vi "VMI_acquire_rewrite_get_loop_working.vi"(4 "Big_image Array":i16[][][](array[numeric]), 5 "Peak Find Settings":T2, 6 "Collect_refs":T1, 7 "Queue Array":T4[](array[typedef]), 8 "error in":errorcluster, 9 "Collection Information":T3[](array[typedef]), 10 "Camera Session":T5, 11 "IMAQ In":T6) -> (0 "error IO":errorcluster, 2 "Peak Array":cluster{"X":sgl, "Y":sgl}[][](array[cluster]), 3 "Histogram":i32[][](array[numeric]))   [LabVIEW 2015]
uses:
  <vilib>/vision/Image Controls.llb/IMAQ Image.ctl
  <vilib>/userdefined/High Color/IMAQdx.ctl
  Type defs/FileAcq_v1_Ctrl.ctl
  Type defs/VMI_collection_refs.ctl
  Array_subVIs/Merge_into_Array.vi
  Array_subVIs/Merge_into_Array_cluster.vi
panel:
  out "xaxis":i32[][](array[numeric])
  out "XY Graph":cluster{"Y":dbl[], "Y":dbl[]}[](graph)
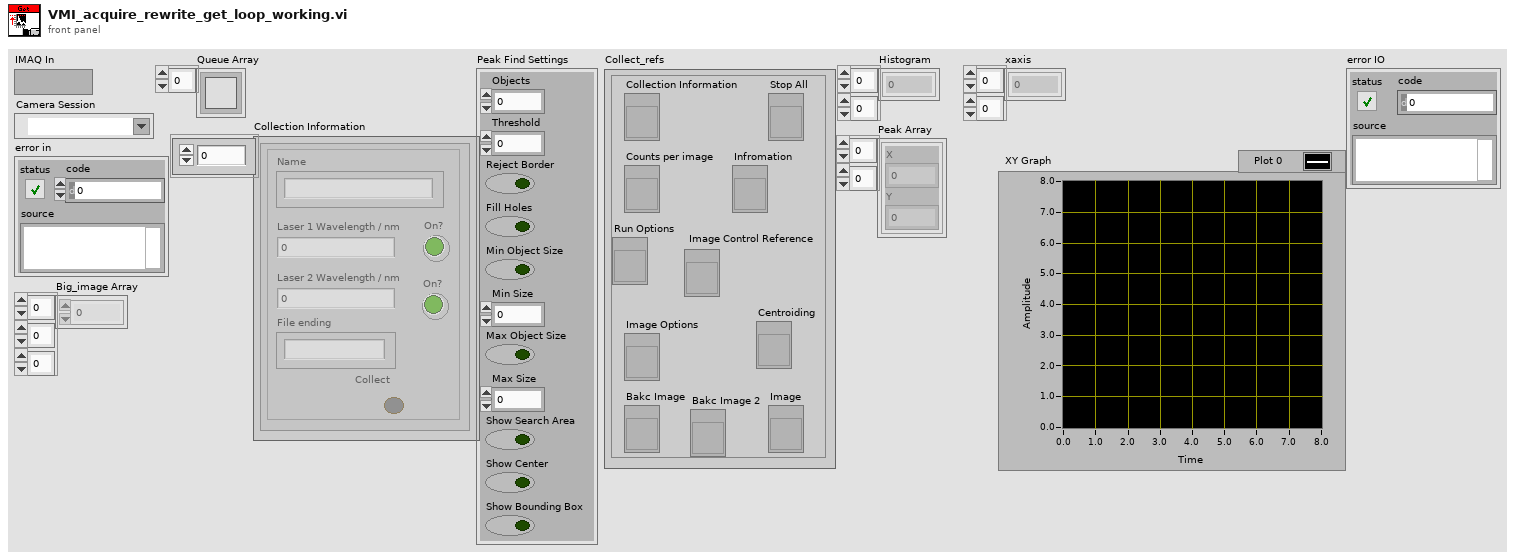
[diagram p1: front panel]
types:
  T1 = typedef "VMI_collection_refs.ctl" = cluster{"Stop All":refnum<vi>, "Collection Information ":refnum<vi>, "Infromation":refnum<vi>, "Counts per image":refnum<vi>, " Image Control Reference ":refnum<vi>, "Run Options":refnum<vi>, "Image Options":refnum<vi>, "Centroiding":refnum<vi>, "Image":refnum<vi>, "Bakc Image":refnum<vi>, "Bakc Image 2":refnum<vi>}
  T2 = cluster{"Objects":u16, "Threshold":i32, "Reject Border":bool, "Fill Holes":bool, "Min Object Size":bool, "Min Size":i32, "Max Object Size":bool, "Max Size":i32, "Show Search Area":bool, "Show Center":bool, "Show Bounding Box":bool}
  T3 = typedef "FileAcq_v1_Ctrl.ctl" = cluster{"Type":string, "LaserWave1":dbl, "Shutter1":bool, "LaserWave2":dbl, "Shutter2":bool, "FileEnd":string, "Collect":bool}
  T4 = typedef "Queue RefNum" = refnum<k1>
  T5 = typedef "IMAQdx.ctl" = refnum<k21>
  T6 = typedef "IMAQ Image.ctl" = refnum<image>
  T7 = cluster{"Total Time / ms":dbl, "Image Total Collection Time":dbl, "Image Loop time / ms":dbl, "Peak Total Find Time":dbl, "Peak Find Time / ms":dbl, "Camera Rate / Hz":dbl, "Total Number of Loops":dbl, "Current Loop Number":dbl, "Number of Image Loops":dbl, "Run Mode":dbl}
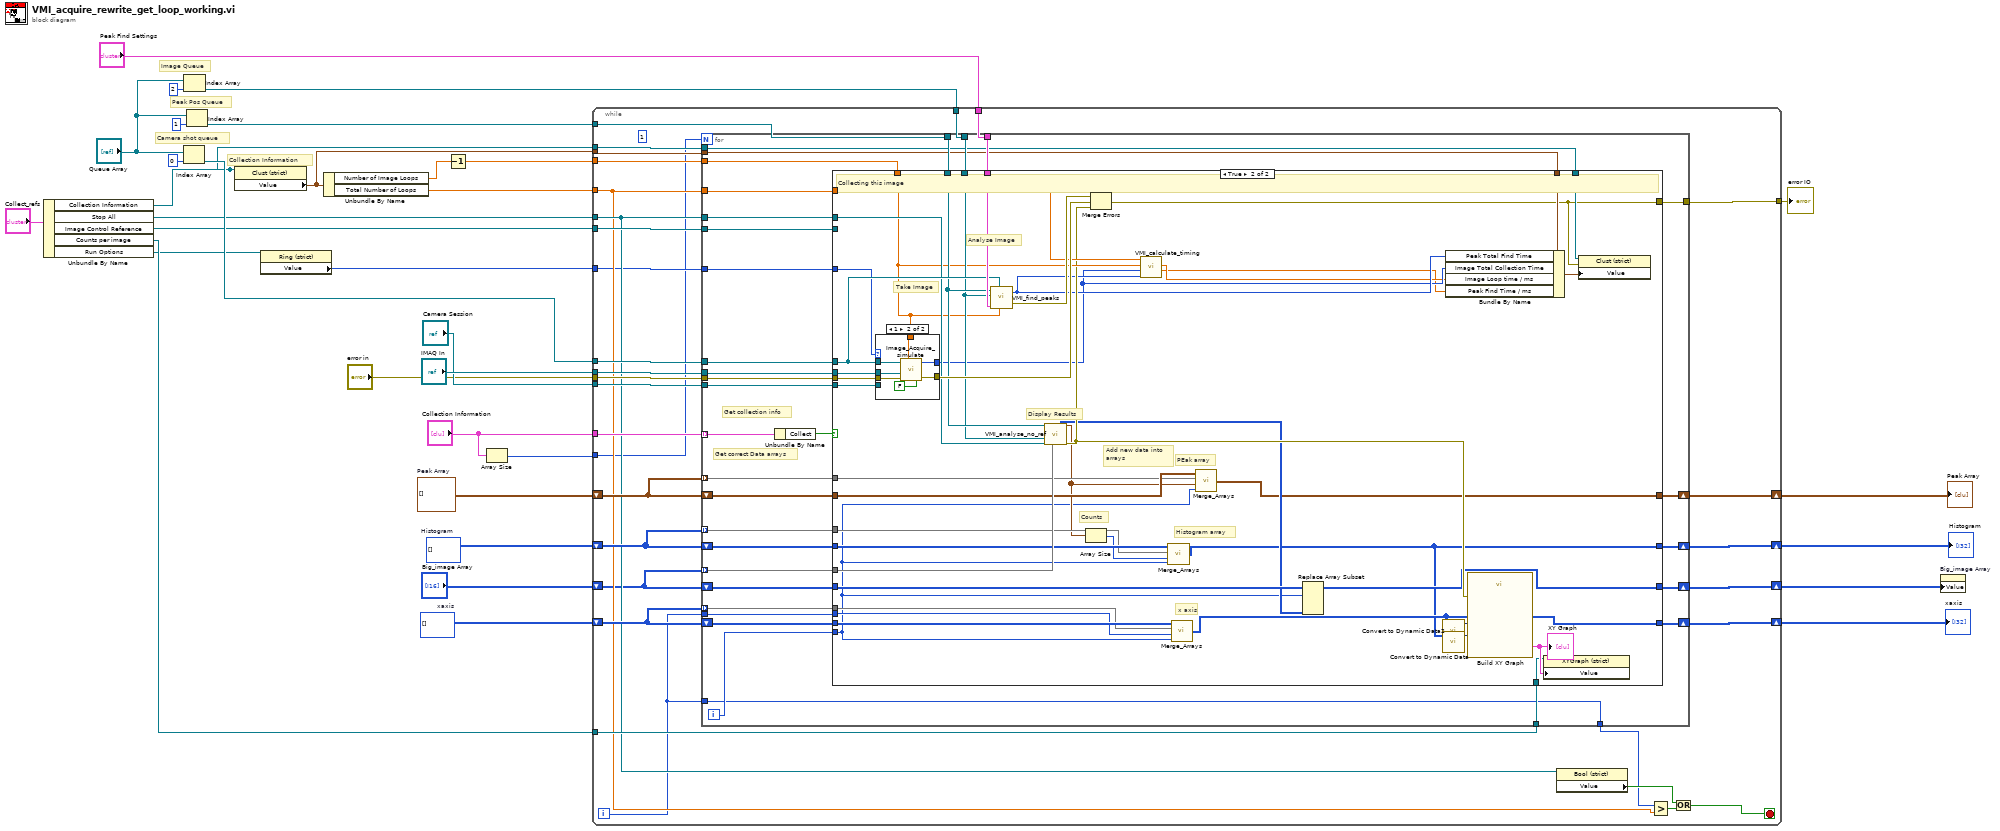
[diagram p0: block diagram]
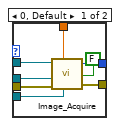
[diagram p3: hidden frame]
diagram:
  w11 = i32[][] []  # xaxis
  w9 = i32[][] []  # Histogram
  w12 = cluster{"X":sgl, "Y":sgl}[][] []  # Peak Array
  # "Collection Information"
  # "Image Queue"
  # "Peak Pos Queue"
  # "Camera shot queue"
  n1 = Unbundle By Name("Collect_refs") -> ("Collection Information"=w14:refnum<vi>, "Stop All"=w20:refnum<vi>, "Image Control Reference"=w19:refnum<vi>, "Counts per image"=w10:refnum<vi>, "Run Options"=w2:refnum<vi>)
  n2 = Index Array(array="Queue Array", index=0) -> (element=w29:T4)
  n3 = Index Array(array="Queue Array", index=2) -> (element=w22:T4)
  n4 = Index Array(array="Queue Array", index=1) -> (element=w25:T4)
  n5 = property class="Clust (strict)"(reference=w14) -> ("Value"=w15:T7)  [unwired: 1 in, 2 out]
  n6 = property class="Ring (strict)"(reference=w2) -> ("Value"=w1:u16)  [unwired: 1 in, 2 out]
  n7 = Unbundle By Name(w15) -> ("Number of Image Loops"=w18:dbl, "Total Number of Loops"=w16:dbl)
  n8 = Decrement(x=w18) -> (x-1=w17:dbl)
  n9 = Array Size(array="Collection Information") -> (size(s)=w13:i32)
  n10 = while {
    tunnel: "IMAQ In" -> [w64]
    tunnel: "Camera Session" -> [w63]
    tunnel: "error in" -> [w62]
    tunnel: w29 -> [w61]
    tunnel: "Collection Information" -> [w60]
    tunnel: "Peak Find Settings" -> [w59]
    tunnel: w25 -> [w58]
    tunnel: w22 -> [w57]
    tunnel: w20 -> [w45]
    tunnel: w19 -> [w56]
    tunnel: w17 -> [w55]
    tunnel: w16 -> [w42]
    tunnel: w15 -> [w54]
    tunnel: w14 -> [w53]
    tunnel: w13 -> [w36]
    tunnel: w10 -> [w50]
    shift-right: [w49] -> w3
    shift-left: w12 -> [w52]
    shift-right: [w47] -> w4
    shift-left: w9 -> [w48]
    shift-right: [w46] -> w8
    shift-left: w11 -> [w51]
    tunnel: [w41] -> w7
    shift-right: [w40] -> w5
    shift-left: "Big_image Array" -> [w39]
    tunnel: w1 -> [w38]
    i -> [w35]
    stop <- w37 stop-if-true
    (unwired) 1
    n11 = for {
      N: w36 -> [_]
      tunnel: w64 -> [w97]
      tunnel: w63 -> [w96]
      tunnel: w62 -> [w95]
      tunnel: w61 -> [w94]
      tunnel: w60 -> [w76] mode=indexing
      tunnel: w59 -> [w92]
      tunnel: w58 -> [w91]
      tunnel: w57 -> [w90]
      tunnel: w45 -> [w89]
      tunnel: w56 -> [w88]
      tunnel: w52 -> [w80] mode=indexing
      tunnel: w55 -> [w86]
      tunnel: w42 -> [w85]
      tunnel: w35 -> [w77]
      tunnel: w51 -> [w78] mode=indexing
      tunnel: w54 -> [w84]
      tunnel: w53 -> [w83]
      tunnel: w48 -> [w79] mode=indexing
      tunnel: w50 -> [w74]
      shift-right: [w73] -> w49
      shift-left: w52 -> [w82]
      shift-right: [w87] -> w47
      shift-left: w48 -> [w72]
      shift-right: [w71] -> w46
      shift-left: w51 -> [w81]
      tunnel: [w70] -> w41
      shift-right: [w68] -> w40
      shift-left: w39 -> [w69]
      tunnel: w39 -> [w67] mode=indexing
      tunnel: w38 -> [w66]
      tunnel: [w65] -> w34
      tunnel: w35 -> [w65]
      i -> [w75]
      # "Get collection info"
      # "Get correct Data arrays"
      # "This loop collects for each required image"
      n12 = Unbundle By Name(w76) -> ("Collect"=w93:bool)
      n13 = case shown="True" w93 {
        tunnel: w97 -> [_ w145]
        tunnel: w96 -> [_ w144]
        tunnel: w95 -> [w102 w143]
        tunnel: w94 -> [_ w141]
        tunnel: w92 -> [_ w142]
        tunnel: w91 -> [_ w138]
        tunnel: w90 -> [_ w137]
        tunnel: w89 -> [_ w136]
        tunnel: w88 -> [_ _]
        tunnel: [w102 w123] -> w70
        tunnel: w80 -> [_ w107]
        tunnel: w82 -> [w101 w108]
        tunnel: [w101 w104] -> w73
        tunnel: w72 -> [w100 w112]
        tunnel: w79 -> [_ w111]
        tunnel: [w100 w109] -> w87
        tunnel: w86 -> [_ w134]
        tunnel: w85 -> [_ w135]
        tunnel: w77 -> [_ w114]
        tunnel: w78 -> [_ w115]
        tunnel: w81 -> [w99 w116]
        tunnel: [w99 w113] -> w71
        tunnel: w84 -> [_ w130]
        tunnel: w83 -> [_ w124]
        tunnel: w75 -> [_ w105]
        tunnel: w74 -> [_ w121]
        tunnel: w69 -> [w98 w119]
        tunnel: [w98 w118] -> w68
        tunnel: w67 -> [_ w120]
        tunnel: w66 -> [_ w103]
        frame False {
          # "Not collecting this image"
        }
        frame True {
          # "x axis"
          # "Histogram array"
          # "PEak array"
          # "Counts"
          # "Add new data into\narrays"
          # "Display Results"
          # "Analyse Image"
          # "Take Image"
          # "Collecting this image"
          n14 = case shown="1" w103 {
            tunnel: w145 -> [w152 w156]
            tunnel: w144 -> [w151 _]
            tunnel: w143 -> [w150 w160]
            tunnel: w141 -> [w149 w155]
            tunnel: [w148 w159] -> w139
            tunnel: w134 -> [w147 w157]
            tunnel: [w146 w158] -> w128
            frame 0, Default {
              n15 = call "Image_Acquire.vi"("Queue Ref in"=w149, "Acquire Time"=w147, "Image Out"=w152, "Session In"=w151, "error in (no error)"=w150, "Test Timing"=FALSE) -> ("Loop Time Out"=w146:i64, "error out"=w148:errorcluster)  [unwired: 1 in]
            }
            frame 1 {
              n16 = call "Image_Acquire_simulate.vi"("Queue Ref in"=w155, "Acquire Time"=w157, "Image Out"=w156, "error in (no error)"=w160, "Test Timing"=FALSE) -> ("Loop Time Out"=w158:i64, "error out"=w159:errorcluster)  [unwired: 2 in]
            }
          }
          n17 = call "VMI_find_peaks.vi"("Acquire Time"=w134, "Acquire Queue In"=w141, "Peak Find Settings"=w142, "Image Queue in"=w137, "Peak Position Queue in"=w138) -> ("error out"=w140:errorcluster, "x-y"=w129:u32)  [unwired: 1 in]
          n18 = call "VMI_analyse_no_ref.vi"("Peak Position Queue in"=w138, "Image in"=w137, "Stop Button Ref"=w136, "Image_array"=w120) -> ("Image_array out"=w117:i32[][], "Peaks Position Out"=w106:cluster{"X":sgl, "Y":sgl}[], "error out"=w132:errorcluster)  [unwired: 7 in, 2 out]
          n19 = Array Size(array=w106) -> (size(s)=w110:i32)
          n20 = Merge Errors(w140, w139, w132) -> (w123:errorcluster)
          n21 = call "VMI_calculate_timing.vi"("Peakfind total time"=w129, "Camera_Total_loop time"=w128, "Number of image loops"=w134, "Total loop Number"=w135) -> ("AveragePeak find time"=w126:dbl, "Average Image Loop time"=w127:dbl)  [unwired: 1 in, 1 out]
          n22 = call-poly "Merge_Arrays.vi"("Index"=w105, "Insert"=w110, "1D Array"=w111, "2D Array"=w112) -> ("Output Array"=w109:i32[][])
          n23 = call-poly "Merge_Arrays.vi"("Index"=w105, "Insert"=w114, "1D Array"=w115, "2D Array"=w116) -> ("Output Array"=w113:i32[][])
          n24 = call-poly "Merge_Arrays.vi"("Index"=w105, "1D Array Insert"=w106, "1D Array"=w107, "2D Array"=w108) -> ("Output Array"=w104:cluster{"X":sgl, "Y":sgl}[][])
          n25 = Replace Array Subset(array=w119, new element=w117, index (dim 0)=w105) -> (w118:i16[][][])  [unwired: 2 in]
          n26 = call "Convert to Dynamic Data2"("2D Array"=w113) -> ("Dynamic Data Type"=w131:dynamicdata)  [unwired: 3 in]
          n27 = call "Convert to Dynamic Data"("2D Array"=w109) -> ("Dynamic Data Type"=w133:dynamicdata)  [unwired: 3 in]
          n28 = Bundle By Name(cluster=w130, "Peak Total Find Time"=w129, "Image Total Collection Time"=w128, "Image Loop time / ms"=w127, "Peak Find Time / ms"=w126) -> (w125:T7)
          n29 = call "Build XY Graph"("error in (no error)"=w132, "Y Input"=w133, "X Input"=w131) -> ("XY Graph"=w122:cluster{"X":dbl[], "Y":dbl[]}[])  [unwired: 7 in, 1 out]
          "XY Graph" <- w122
          n30 = property on="Property Node" class="XYGraph (strict)"(reference=w121, "Value"=w122) -> ()  [unwired: 1 in, 2 out]
          n31 = property class="Clust (strict)"(reference=w124, error in=w123, "Value"=w125) -> ()  [unwired: 2 out]
        }
      }
    }
    n32 = property on="Property Node" class="Bool (strict)"(reference=w45) -> ("Value"=w44:bool)  [unwired: 1 in, 2 out]
    n33 = Greater?(x=w34, y=w42) -> (0:w43:bool)
    n34 = Or(x=w44, y=w43) -> (x .or. y?=w37:bool)
  }
  "Histogram" <- w4
  "Peak Array" <- w3
  "xaxis" <- w8
  "error IO" <- w7
  n35 = property on="Big_image Array" class="Arr (strict)"("Value"=w5) -> ()  [unwired: 2 in, 2 out]
